vi "Bar100GetCalibration.vi"() -> ()   [LabVIEW 2021]
uses:
  <vilib>/myRIO/Instrument Drivers/Onboard IO/I2C/typedefs/I2C User Configuration.ctl
  <vilib>/myRIO/Instrument Drivers/Onboard IO/I2C/typedefs/I2C Transfer Rate.ctl
  <vilib>/myRIO/Instrument Drivers/Onboard IO/I2C/typedefs/I2C Reference.ctl
  <vilib>/myRIO/Common/Instrument Driver Framework/Utilities/typedefs/myRIO Generic Hardware Reference.ctl
  <vilib>/myRIO/Common/Instrument Driver Framework/Utilities/typedefs/Hardware Version Enum.ctl
  <vilib>/myRIO/Common/Instrument Driver Framework/Utilities/typedefs/myRIO v1.0 Reference.ctl
  <vilib>/myRIO/Common/Instrument Driver Framework/Utilities/typedefs/Generic FPGA Reference.ctl
  <vilib>/myRIO/Common/Instrument Driver Framework/myRIO v1.0/I2C/typedefs/I2C Channels Enum.ctl
  <vilib>/myRIO/Instrument Drivers/Onboard IO/I2C/typedefs/I2C Configuration.ctl
  <vilib>/userDefined/High Color/nirio_resource_hc.ctl
  <vilib>/myRIO/Common/Instrument Driver Framework/myRIO v1.0/I2C/vis/myRIO v1.1 Open I2C.vi
  <vilib>/myRIO/Common/Instrument Driver Framework/Utilities/vis/Validate Channels.vi
  <vilib>/myRIO/Common/Instrument Driver Framework/myRIO v1.0/I2C/vis/myRIO v1.0 Reserve I2C.vi
  <vilib>/myRIO/Common/Instrument Driver Framework/myRIO v1.0/I2C/vis/myRIO v1.0 Close I2C.vi
  <vilib>/myRIO/Common/Instrument Driver Framework/myRIO v1.0/I2C/vis/myRIO v1.0 Build MUX Configuration I2C.vi
  <vilib>/myRIO/Common/Instrument Driver Framework/myRIO v1.0/Resource Manager/vis/myRIO v1.0 Reserve Channel List.vi
  <vilib>/myRIO/Common/Instrument Driver Framework/myRIO v1.0/I2C/vis/myRIO v1.0 Unreserve I2C.vi
  <vilib>/myRIO/Common/Instrument Driver Framework/myRIO v1.0/Resource Manager/vis/myRIO v1.0 Create Configuration List.vi
  <vilib>/myRIO/Common/Instrument Driver Framework/myRIO v1.0/Resource Manager/vis/myRIO v1.0 Reserve Channel.vi
  <vilib>/myRIO/Common/Instrument Driver Framework/myRIO v1.0/Resource Manager/vis/myRIO v1.0 Unreserve Channel.vi
  <vilib>/myRIO/Common/Instrument Driver Framework/myRIO v1.0/Resource Manager/vis/myRIO v1.0 Unreserve Channel List.vi
  <vilib>/myRIO/Common/Instrument Driver Framework/myRIO v1.0/Resource Manager/vis/myRIO v1.0 Build Mutex Name.vi
  <vilib>/Utility/VariantDataType/GetNumericInfo.vi
  <vilib>/Utility/error.llb/Error Cluster From Error Code.vi
  <vilib>/myRIO/Common/Instrument Driver Framework/myRIO v1.0/myRIO v1.1 Open.vi
  <vilib>/myRIO/Common/Instrument Driver Framework/Utilities/vis/IO Manager.vi
  <vilib>/myRIO/Common/Instrument Driver Framework/Utilities/vis/Configuration Manager.vi
  <vilib>/myRIO/Common/Instrument Driver Framework/myRIO v1.0/Resource Manager/vis/myRIO v1.0 Configure IO.vi
  <vilib>/myRIO/Common/Instrument Driver Framework/myRIO v1.0/myRIO v1.0 Close.vi
  <vilib>/myRIO/Common/Instrument Driver Framework/myRIO v1.0/I2C/vis/myRIO v1.0 Configure I2C.vi
  <vilib>/myRIO/Common/Instrument Driver Framework/myRIO v1.0/I2C/vis/myRIO v1.0 Write I2C.vi
  <vilib>/myRIO/Common/Instrument Driver Framework/myRIO v1.0/I2C/vis/myRIO v1.0 Read I2C.vi
  <vilib>/myRIO/Common/Instrument Driver Framework/myRIO v1.0/I2C/vis/myRIO v1.0 Shutdown I2C.vi
  <vilib>/myRIO/Instrument Drivers/Onboard IO/I2C/vis/myRIO I2C Open.xnode
  <vilib>/myRIO/Instrument Drivers/Onboard IO/I2C/I2C.lvlib
panel:
  out "mode":u32
  out "P_mode":dbl
  out "P_max":dbl
  out "P_min":dbl
  out "error out":errorcluster
  in  "error in (no error)":errorcluster
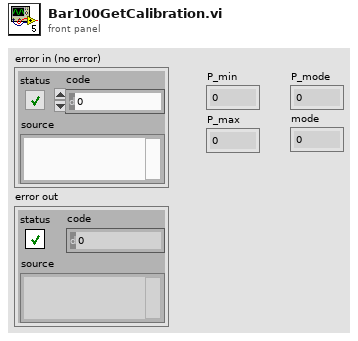
[diagram p1: front panel]
types:
  T1 = typedef "I2C.lvlib/I2C User Configuration.ctl" = cluster{"I2C Transfer Rate":T2}
  T2 = typedef "I2C.lvlib/I2C Transfer Rate.ctl" = enum16{"Standard mode (100 kbps)", "Fast mode (400 kbps)"}
  T3 = typedef "I2C.lvlib/I2C Reference.ctl" = cluster{"myRIO Reference":T4, "I2C Channels Enum":T8, "I2C Configuration":T9}
  T4 = typedef "myRIO Generic Hardware Reference.ctl" = cluster{"myRIO Model":T5, "myRIO Hardware Reference":T6}
  T5 = typedef "Hardware Version Enum.ctl" = enum16{"Unknown", "myRIO-1900", "myRIO-1950", "roboRIO", "NI ELVIS RIO CM", "ELVIS III"}
  T6 = typedef "myRIO v1.0 Reference.ctl" = cluster{"Generic FPGA Reference":T7, "Allow multiple opens":bool}
  T7 = typedef "Generic FPGA Reference.ctl" = refnum<k20>
  T8 = typedef "I2C Channels Enum.ctl" = enum16{"Not Connected", "A/I2C", "B/I2C", "I2C/I2C"}
  T9 = typedef "I2C.lvlib/I2C Configuration.ctl" = cluster{"I2C Transfer Rate":T2}
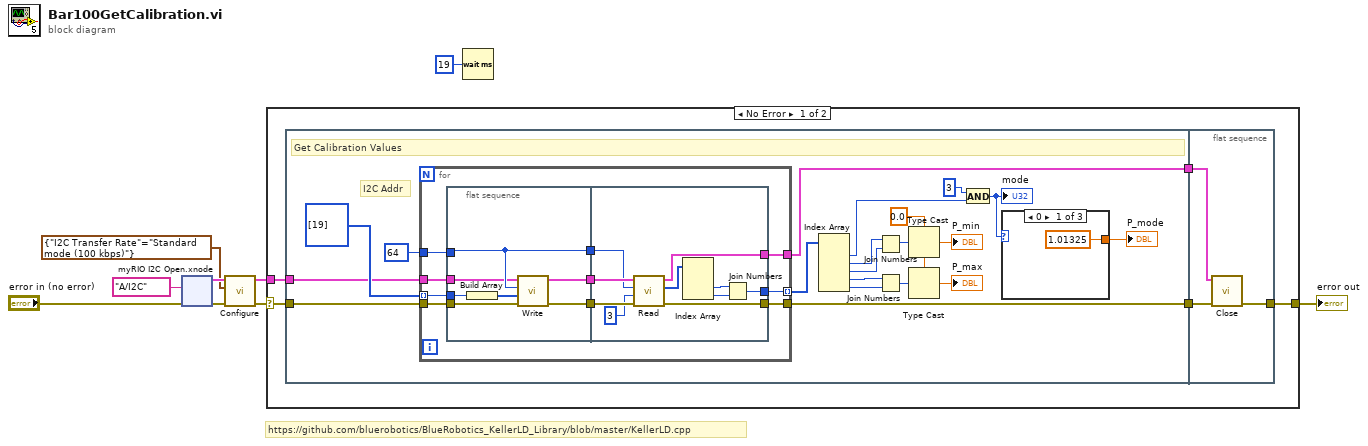
[diagram p0: block diagram]
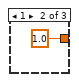
[diagram p2: hidden frame]
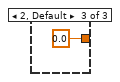
[diagram p3: hidden frame]
diagram:
  # "https://github.com/bluerobotics/BlueRobotics_KellerLD_Library/blob/master/KellerLD.cpp"
  n1 = xnode "myRIO I2C Open.xnode"("error in (no error)"="error in (no error)", "Channel Name"=tag "A/I2C") -> ("error out"=w7:errorcluster, "I2C Ref Out"=w6:T3)  [unwired: 1 in]
  n2 = call <vilib>:"Configure.vi"("error in (no error)"=w7, "I2C User Configuration"=T1 {"I2C Transfer Rate"=enum."Standard mode (100 kbps)"}, "I2C Ref In"=w6) -> ("error out"=w8:errorcluster, "I2C Ref Out"=w9:T3)  [unwired: 7 in]
  n3 = case shown="No Error" w8 {
    selector: w8 -> [w13 w68]
    tunnel: w9 -> [w14 _]
    tunnel: [w10 w68] -> w2
    frame No Error {
      n4 = flat-sequence {
        tunnel: [w32] -> w12
        tunnel: [w31] -> w11
        tunnel: w14 -> [w15]
        tunnel: w13 -> [w16]
        tunnel: w12 -> [w67]
        tunnel: w11 -> [w66]
        tunnel: [w65] -> w10
        frame #0 {
          w17 = 0.0
          # "I2C Addr"
          # "Get Calibration Values"
          n5 = for {
            tunnel: w15 -> [w47]
            tunnel: w16 -> [w46]
            tunnel: u8[] [19] ("Bytes to Write") -> [w44] mode=indexing
            tunnel: u8 64 ("Slave Address (7-bit)") -> [w45]
            tunnel: [w43] -> w32
            tunnel: [w42] -> w31
            tunnel: [w41] -> w30 mode=indexing
            n6 = flat-sequence {
              tunnel: w44 -> [w53]
              tunnel: w45 -> [w54]
              tunnel: w46 -> [w51]
              tunnel: w47 -> [w49]
              tunnel: [w48] -> w40
              tunnel: [w50] -> w39
              tunnel: [w54] -> w38
              tunnel: [w61] -> w43
              tunnel: [w60] -> w42
              tunnel: [w56] -> w41
              tunnel: w40 -> [w64]
              tunnel: w39 -> [w63]
              tunnel: w38 -> [w55]
              frame #0 {
                n7 = Build Array(w53) -> (w52:u8[])
                n8 = call <vilib>:"Write.vi"("error in (no error)"=w51, "Bytes to Write"=w52, "Slave Address (7-bit)"=w54, "I2C Ref In"=w49) -> ("error out"=w50:errorcluster, "I2C Ref Out"=w48:T3)  [unwired: 6 in]
              }
              frame #1 {
                n9 = call <vilib>:"Read.vi"("error in (no error)"=w63, "Byte Count"=u32 3, "Slave Address (7-bit)"=w55, "I2C Ref In"=w64) -> ("error out"=w60:errorcluster, "Bytes Read"=w59:u8[], "I2C Ref Out"=w61:T3)  [unwired: 4 in]
                n10 = Index Array(array=w59) -> (element #2=w58:u8, element #3=w57:u8)  [unwired: 3 in, 1 out]
                n11 = Join Numbers(hi=w58, lo=w57) -> ((hi.lo)=w56:u16)
              }
            }
          }
          n12 = Index Array(array=w30) -> (element #1=w26:u16, element #2=w25:u16, element #3=w24:u16, element #4=w23:u16, element #5=w22:u16)  [unwired: 5 in]
          n13 = Join Numbers(hi=w25, lo=w24) -> ((hi.lo)=w21:u32)
          n14 = Join Numbers(hi=w23, lo=w22) -> ((hi.lo)=w19:u32)
          n15 = Type Cast(type=w17, x=w21) -> (*(type *) &x=→"P_min":dbl)
          n16 = Type Cast(type=w17, x=w19) -> (*(type *) &x=→"P_max":dbl)
          n17 = And(x=u32 3, y=w26) -> (x .and. y?=w28:u32)
          "mode" <- w28
          n18 = case shown="0" w28 {
            tunnel: [1.01325 1.0 0.0] -> w27
            frame 0 {
            }
            frame 1 {
            }
            frame 2, Default {
            }
          }
          "P_mode" <- w27
        }
        frame #1 {
          n19 = call <vilib>:"Close.vi"("error in (no error)"=w66, "I2C Ref In"=w67) -> ("error out"=w65:errorcluster)  [unwired: 9 in]
        }
      }
    }
    frame Error {
    }
  }
  "error out" <- w2
  n20 = Wait (ms)(milliseconds to wait=u32 19) -> ()  [unwired: 1 out]
